vi "Spectral Measurements.vi"(6 "dt":dbl, 8 "DC SHIFT":dbl=-1.764, 9 "Voltage Divider IN":dbl, 10 "Number of samples":dbl, 11 "Array In":dbl[](array[numeric])) -> (0 "Array Out":dbl[](array[numeric]), 1 "Min":dbl, 2 "Max":dbl, 3 "Graph 2":cluster{"f0":dbl, "df":dbl, "magnitude":dbl[]}(graph), 4 "VDC":dbl, 5 "Upper Loc":dbl, 7 "Lower Loc":dbl)   [LabVIEW 2012]
uses:
  <vilib>/express/express analysis/Spectral/Block/exnSpectralBlock spectral measurements peak poly.vi
  <vilib>/express/express analysis/Spectral/Block/exnSpectralBlock spectral measurements peak WFM.vi
  <vilib>/express/express analysis/Spectral/XNode/ExpressSpectralMeasurementsBlockNode.xnode
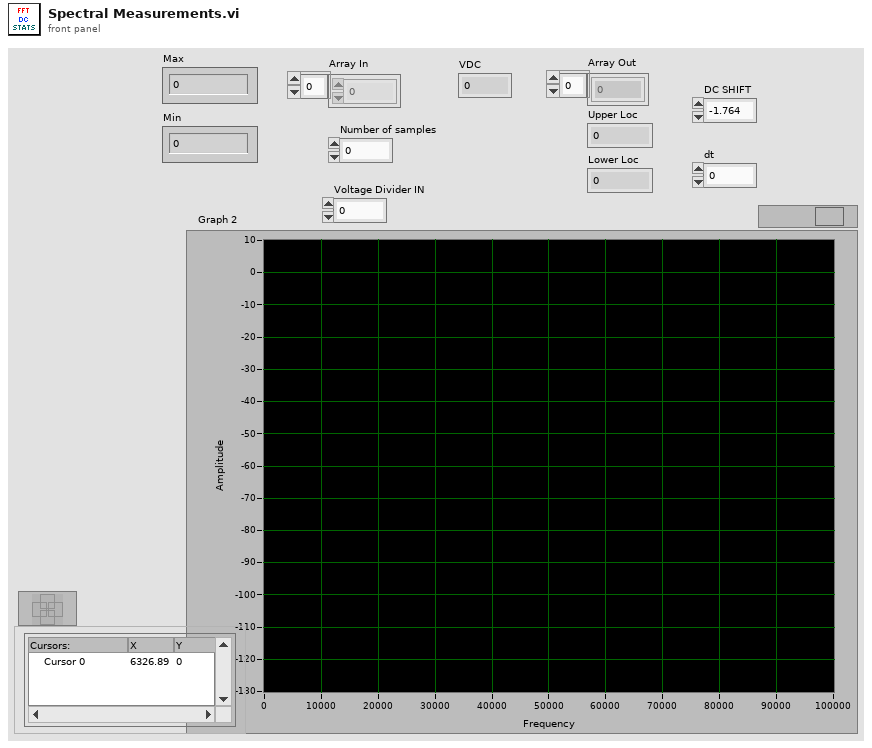
[diagram p1: front panel]
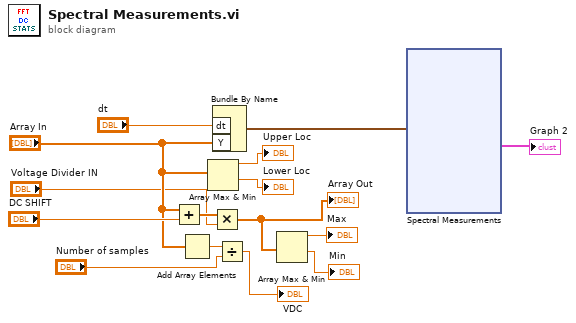
[diagram p0: block diagram]
diagram:
  n1 = Add(x="Array In", y="DC SHIFT") -> (x+y=w11:dbl[])
  n2 = Add Array Elements(numeric array="Array In") -> (sum=w15:dbl)
  n3 = Array Max & Min(array="Array In") -> (max value=→"Upper Loc":dbl, min value=→"Lower Loc":dbl)  [unwired: 2 out]
  n4 = Multiply(x=w11, y="Voltage Divider IN") -> (x*y=w2:dbl[])
  "Array Out" <- w2
  n5 = Bundle By Name("dt"="dt", "Y"="Array In") -> (w9:waveform(dbl))  [unwired: 1 in]
  n6 = Divide(x=w15, y="Number of samples") -> (x/y=→"VDC":dbl)
  n7 = Array Max & Min(array=w2) -> (max value=→"Max":dbl, min value=→"Min":dbl)  [unwired: 2 out]
  n8 = xnode "Spectral Measurements"("Signals"=w9) -> ("FFT - (Peak)"=→"Graph 2":cluster{"f0":dbl, "df":dbl, "magnitude":dbl[]})  [unwired: 1 in, 2 out]
